vi "Set Time Type.vi"(0 "reference in":refnum<class "RPC.lvclass">, 5 "error in (no error)":errorcluster, 7 "Time Type":enum16{"Response", "Drive"}(ring)) -> (14 "reference out":refnum<class "RPC.lvclass">, 19 "error out":errorcluster)   [LabVIEW 2022 SP3, in "RPC.lvclass"]
uses:
  RPC.lvclass
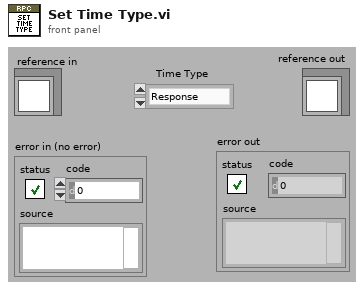
[diagram p1: front panel]
types:
  T1 = typedef "RPC.lvclass/ObjectAttributesRef.ctl" = refnum<data-value>
  T2 = typedef "RPC.lvclass/ObjectAttributes.ctl" = cluster{"File Refnum":refnum<file>, "File total size":i32, "Offset from start of file":i32, "Time Type":enum16{"Response", "Drive"}, "Full Scale":dbl[unit], "New Time Data Obj?":bool, "Header":cluster{"Num Header":i32, "Num Parameter":i32, "Nb Channels":i32, "dT":dbl, "Number of Groups":i32, "Group size":i32, "Units":string[], "Names":string[], "Sensitivity":dbl[], "Complete header":string[]}, "Time Data":refnum<class "GSwFormDSP.lvclass">}
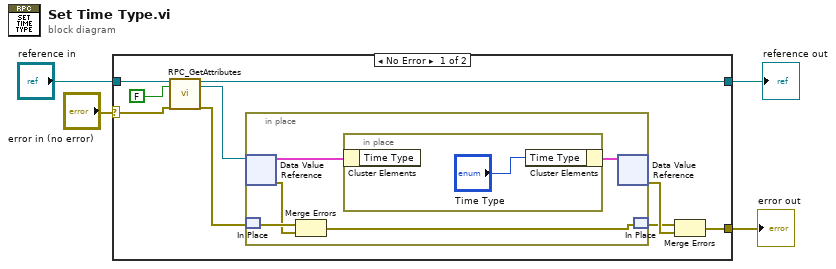
[diagram p0: block diagram]
diagram:
  n1 = case shown="No Error" "error in (no error)" {
    selector: "error in (no error)" -> [w9 w21]
    tunnel: [w13 w21] -> w3
    tunnel: [w8 w20] -> w1
    tunnel: "reference in" -> [w11 w20]
    frame No Error {
      n2 = call "RPC_GetAttributes.vi"("reference in"=w11, "return data? (T)"=FALSE, "error in (no error)"=w9) -> ("reference out"=w8:refnum<class "RPC.lvclass">, "attributes ref"=w7:T1, "error out"=w6:errorcluster)  [unwired: 13 in, 1 out]
      n3 = in-place {
        n4 = in-place-dvr #1(w7) -> (w17:T2, w15:errorcluster)
        n5 = in-place-match #2(w6) -> (w16:errorcluster)
        n6 = Merge Errors(w16, w15) -> (w14:errorcluster)
        n7 = in-place {
          n8 = in-place-cluster #3(w17) -> ()  [unwired: 1 out]
          n9 = in-place-cluster #3("Time Type"="Time Type") -> (w18:T2)
        }
        n10 = in-place-dvr #1(w18) -> (w12:errorcluster)  [unwired: 1 out]
        n11 = in-place-match #2(w14) -> (w5:errorcluster)
      }
      n12 = Merge Errors(w5, w12) -> (w13:errorcluster)
    }
    frame Error {
    }
  }
  "error out" <- w3
  "reference out" <- w1
